vi "wheel arc length.vi"(3 "error in":errorcluster, 5 "FPGA VI Reference In":refnum<k20>) -> (0 "error out":errorcluster, 1 "Right arc in m":dbl, 2 "Left arc in m":dbl)   [LabVIEW 2021]
uses:
  <vilib>/rvi/interface/nirviReadWriteControl/nirviReadWriteControl.xnode
  NiFpgaLv.dll
  <vilib>/Utility/error.llb/Error Cluster From Error Code.vi
  <vilib>/rvi/interface/Simulation/niFpgaSimulationCallBeginRW.vi
  <vilib>/rvi/errors/niLvFpgaAdjustHostInterfaceError.vi
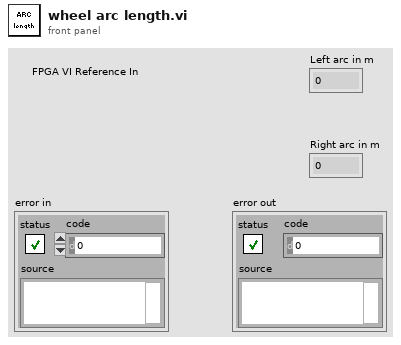
[diagram p1: front panel]
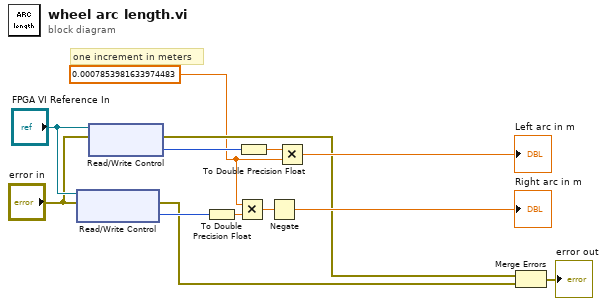
[diagram p0: block diagram]
diagram:
  w1 = 0.0007853981633974483
  # "one increment in meters"
  n1 = xnode "Read/Write Control"("FPGA VI Reference In"="FPGA VI Reference In", "error in"="error in") -> ("error out"=w4:errorcluster, "right counts"=w7:i32)  [unwired: 1 out]
  n2 = xnode "Read/Write Control"("FPGA VI Reference In"="FPGA VI Reference In", "error in"="error in") -> ("error out"=w5:errorcluster, "left counts"=w8:i32)  [unwired: 1 out]
  n3 = To Double Precision Float(number=w7) -> (double precision float=w12:dbl)
  n4 = Multiply(x=w1, y=w12) -> (x*y=w11:dbl)
  n5 = To Double Precision Float(number=w8) -> (double precision float=w13:dbl)
  n6 = Negate(x=w11) -> (-x=→"Right arc in m":dbl)
  n7 = Multiply(x=w13, y=w1) -> (x*y=→"Left arc in m":dbl)
  n8 = Merge Errors(w5, w4) -> (→"error out":errorcluster)
